vi "Contingency Table.vi"(0 "Table":i32[][](array[numeric]) format="%0.0f") -> (1 "x":dbl format="%0.2f", 2 "probability":dbl format="%0.6f", 3 "error":i32)   [LabVIEW 2017, in "NI_AALPro.lvlib"]
doc: "Computes the Pearson 2 test for independence. This function is used to test whether the row and column categorical variables of the contingency table are independent."
uses:
  <vilib>/Analysis/NI_AALPro.lvlib
  <resource>/lvanlys.dll
panel:
  # "Contingency Table"
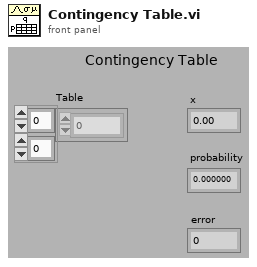
[diagram p1: front panel]
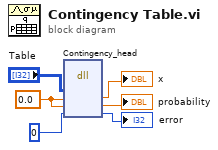
[diagram p0: block diagram]
diagram:
  w4 = 0.0
  n1 = dll-call lib="e:/builds/penguin/labview/branches/2017/dev/dist/resource/lvanlys.*" fn="Contingency_head"("Table"="Table", w4, w4, 0) -> (→"x":dbl, →"probability":dbl, →"error":i32)  [unwired: 5 in, 2 out]
